vi "Read Laser Controller.vi"(8 "error in (no error)":errorcluster, 11 "Laser View in":refnum<class "Laser View.lvclass">) -> (0 "error out":errorcluster, 2 "Laser Controller.lvclass":refnum<class "Laser Controller.lvclass">, 3 "Laser View out":refnum<class "Laser View.lvclass">)   [LabVIEW 2022 SP3]
uses:
  Laser View.lvclass
  C:/XY Stage/iView/base view/base view.lvclass
  C:/XY Stage/iView/iView/iView.lvclass
  C:/XY Stage/Laser/Laser View/Laser View.lvclass
  Laser Controller/Laser Controller.lvclass
  C:/XY Stage/Laser/Laser Controller api/Laser API.lvclass
  C:/XY Stage/Laser/Laser API/Laser.lvclass
  C:/XY Stage/Laser/Get Laser Status/Get Laser Status.lvclass
  C:/XY Stage/Laser/Laser Controller/Laser Controller.lvclass
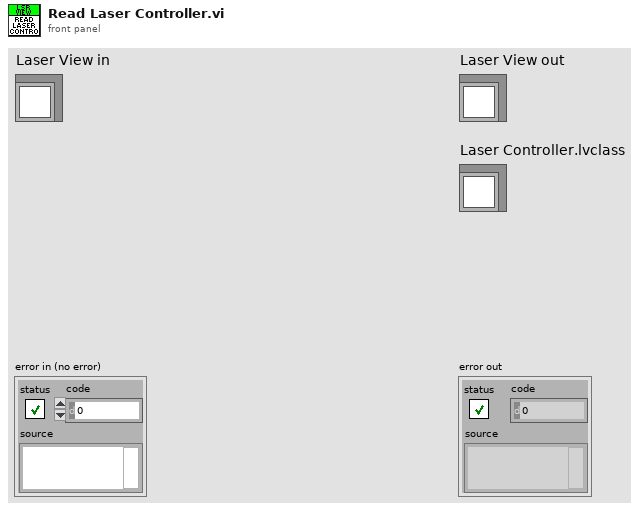
[diagram p1: front panel]
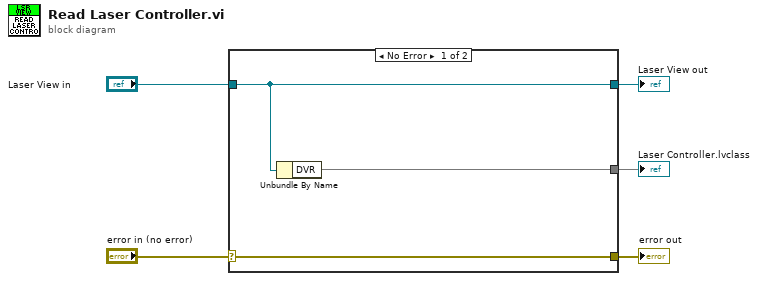
[diagram p0: block diagram]
diagram:
  n1 = case shown="No Error" "error in (no error)" {
    selector: "error in (no error)" -> [w8 w9]
    tunnel: [w8 w9] -> w4
    tunnel: [w7 w10] -> w2
    tunnel: "Laser View in" -> [w7 w10]
    tunnel: [w6 _] -> w1
    frame No Error {
      n2 = Unbundle By Name(w7) -> ("DVR"=w6)
    }
    frame Error {
    }
  }
  "error out" <- w4
  "Laser View out" <- w2
  "Laser Controller.lvclass" <- w1
